vi "古田户外一体站流程质控自动启动.vi"(11 "参数":T1={"是否启用仪器"=FALSE, "CODMn"={"启动测量模式"={"测量模式"=enum."水样测量"}, "确定按钮"=TRUE}, "启动模块"={"氨氮"=FALSE, "总磷"=FALSE, "总氮"=FALSE, "COD"=FALSE}, "常规启动"=FALSE, "直接启动"=FALSE}) -> ()   [LabVIEW 2016, in "质控单元.lvlib"]
uses:
  PLC/PLC.lvlib
panel:
  out "枚举 2":enum16{"初始化", "采配水启动", "等待", "配水", "排水", "结束"}(ring)
  out "枚举":enum16{"初始化", "采配水启动", "等待", "配水", "排水", "结束"}(ring)
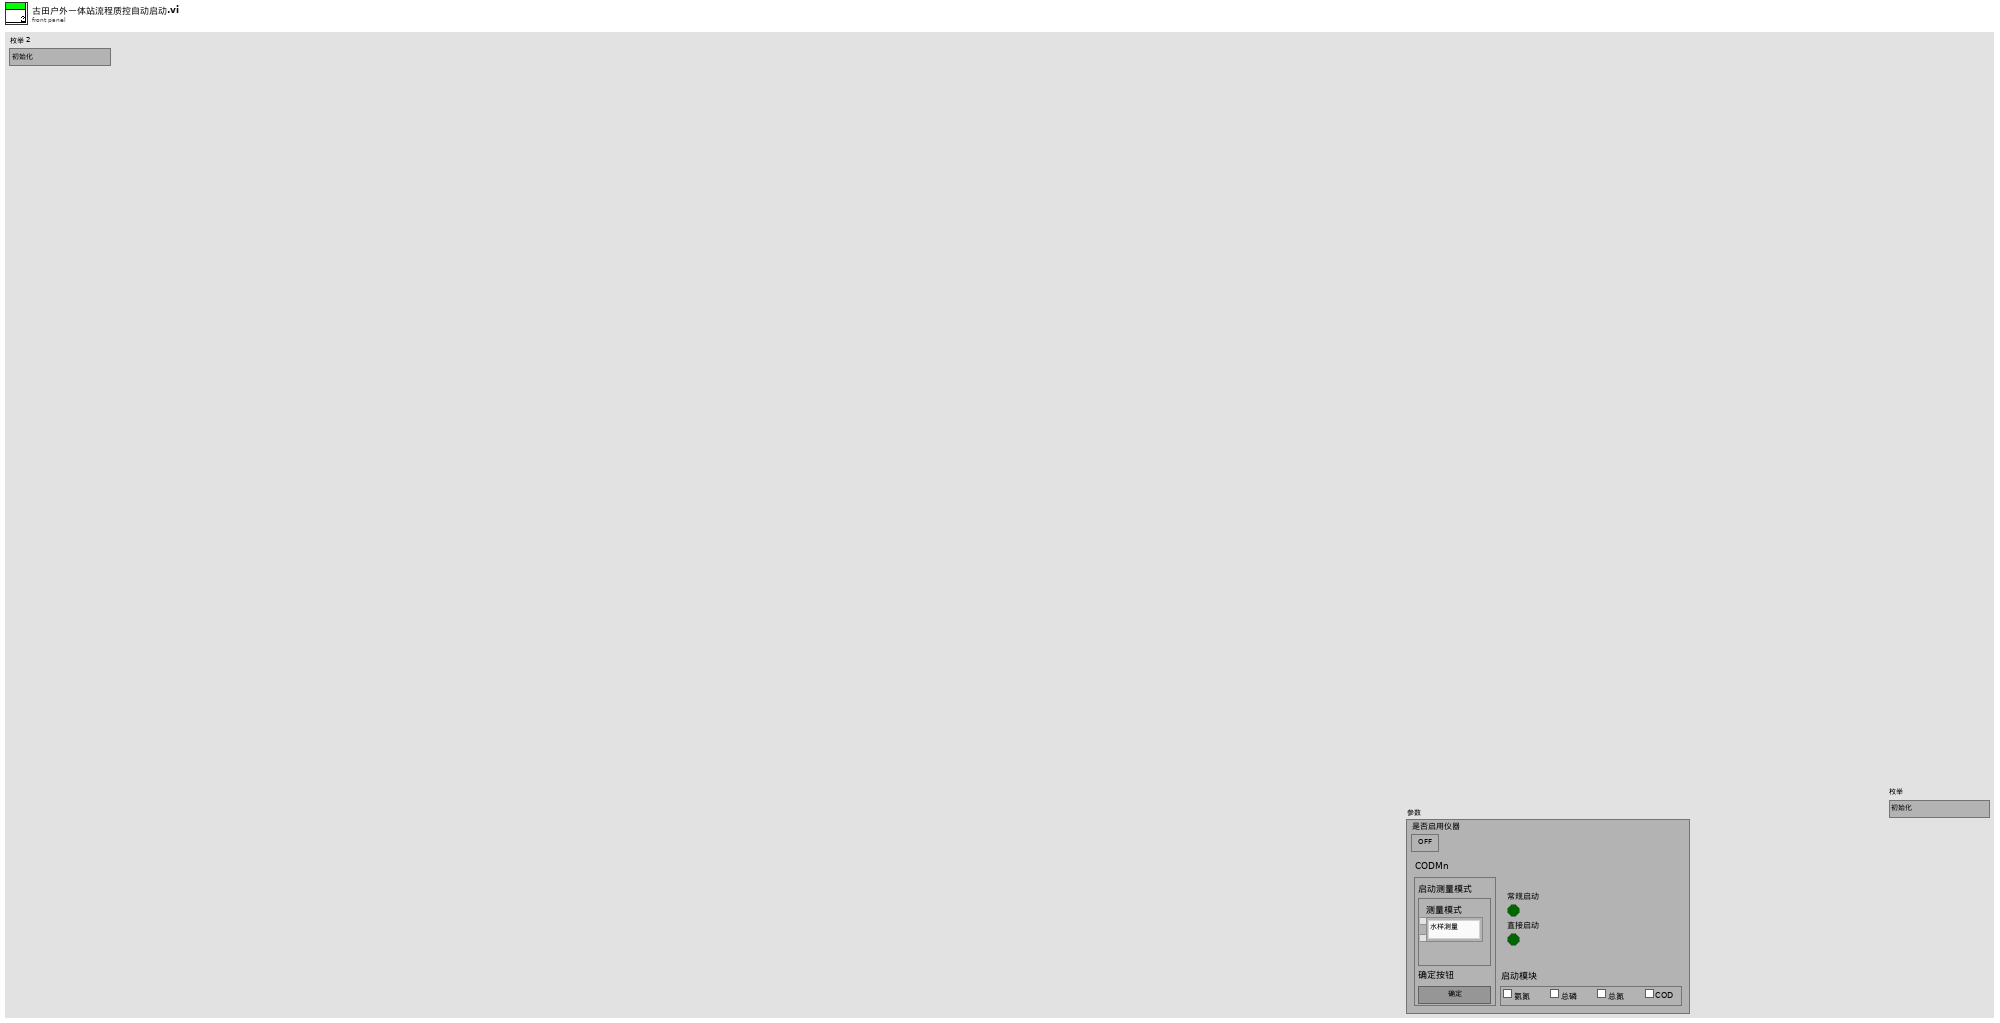
[diagram p1: front panel]
types:
  T1 = cluster{"是否启用仪器":bool, "CODMn":cluster{"启动测量模式":cluster{"测量模式":enum16{"水样测量", "标样核查", "加标回收", "平行样", "校零", "校标"}}, "确定按钮":bool}, "启动模块":cluster{"氨氮":bool, "总磷":bool, "总氮":bool, "COD":bool}, "常规启动":bool, "直接启动":bool}
  T2 = cluster{"命令":string, cluster{"starting address":u16, "holding register value":u16}}
  T3 = cluster{"R0":i16, "R1":i16, "R2":i16, "R3":i16, "R4":i16, "R5":i16, "R6":i16, "R7":i16, "R8":i16, "R9":i16, "R10":i16, "R11":i16, "R12":i16, "R13":i16, "R14":i16, "R15":i16, "R16":i16, "R17":i16, "R18":i16, "R19":i16, "R20":i16, "R21":i16}
  T4 = enum32{"Bad", "Idle", "Run top level", "Running"}
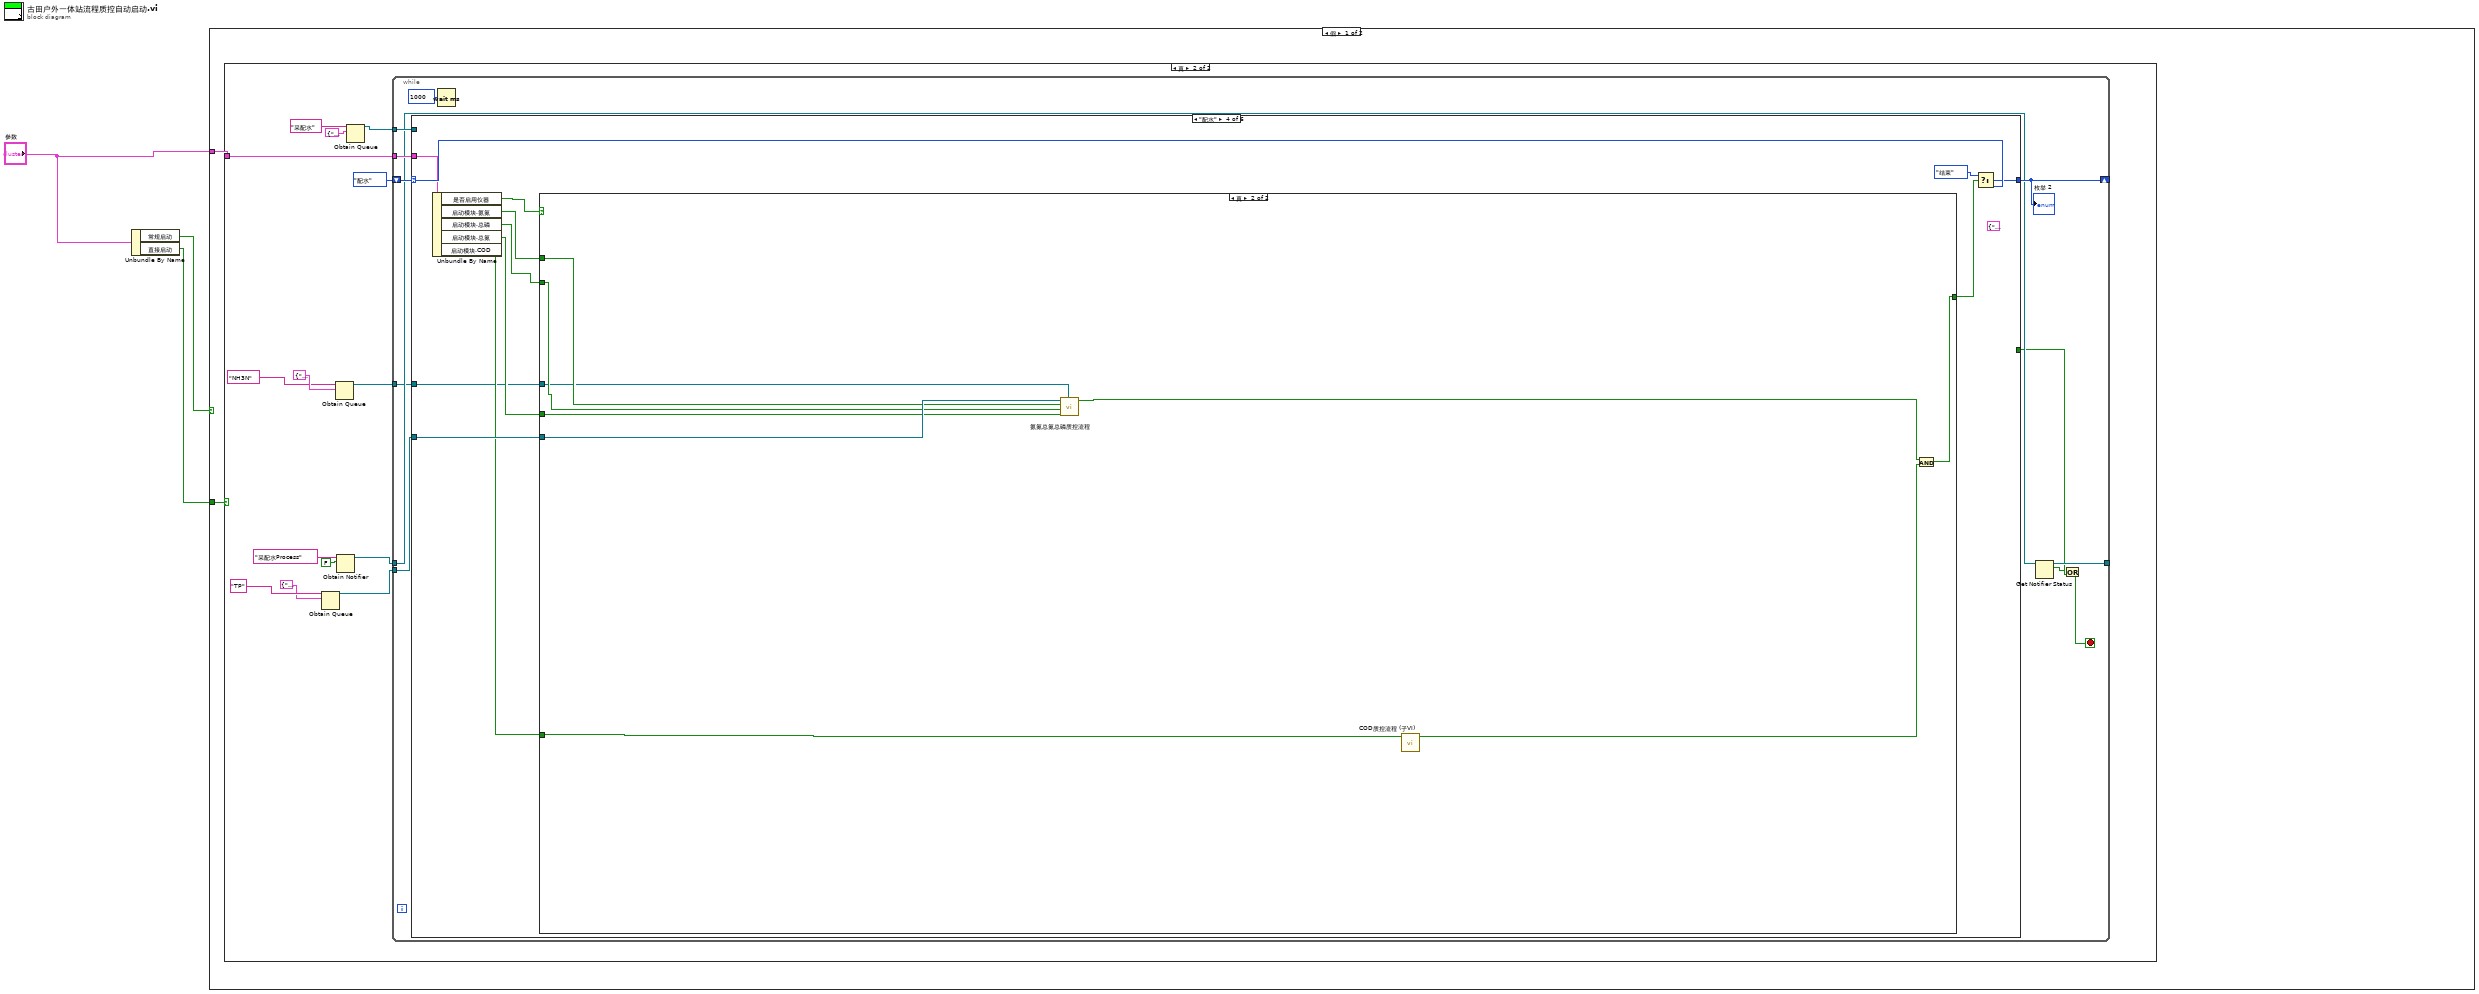
[diagram p0: block diagram]
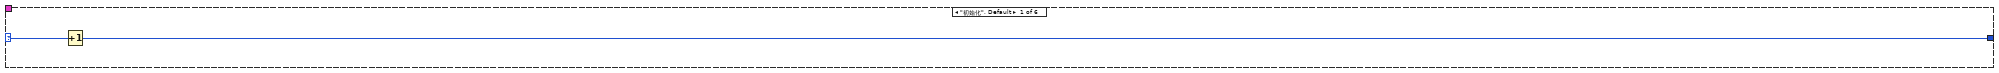
[diagram p3: hidden frame]
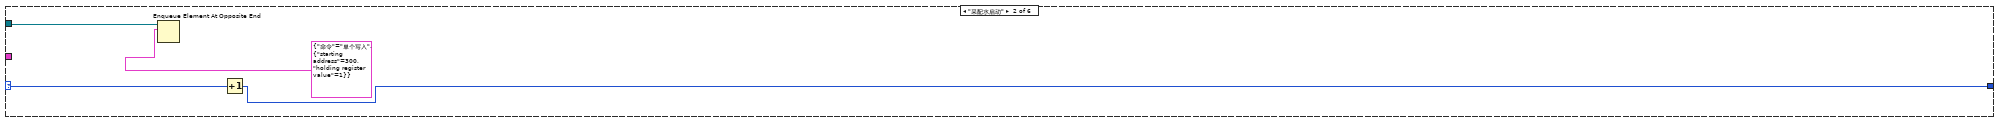
[diagram p4: hidden frame]
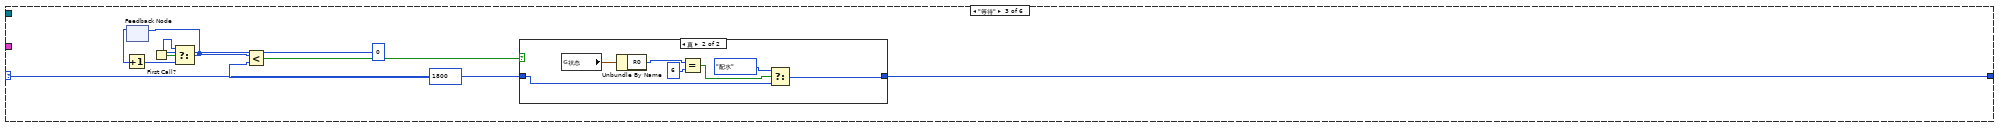
[diagram p5: hidden frame]
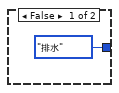
[diagram p6: hidden frame]
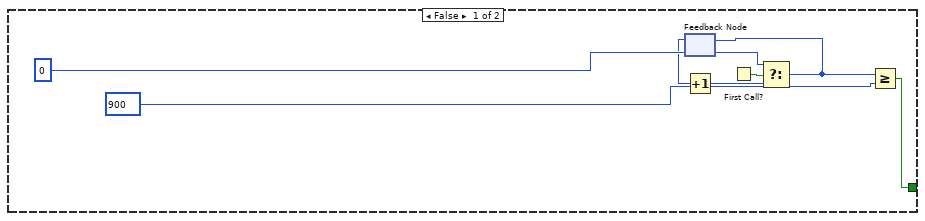
[diagram p7: hidden frame]
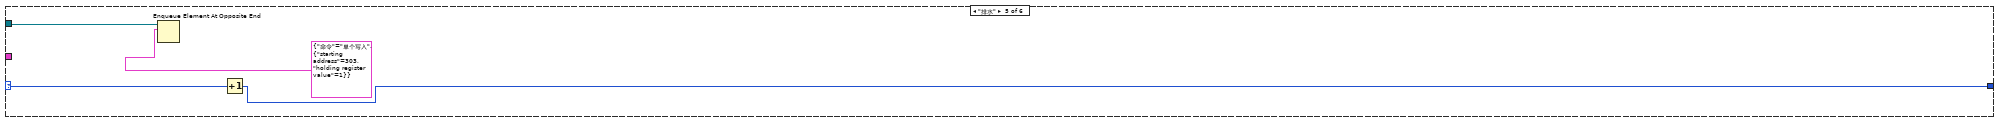
[diagram p8: hidden frame]
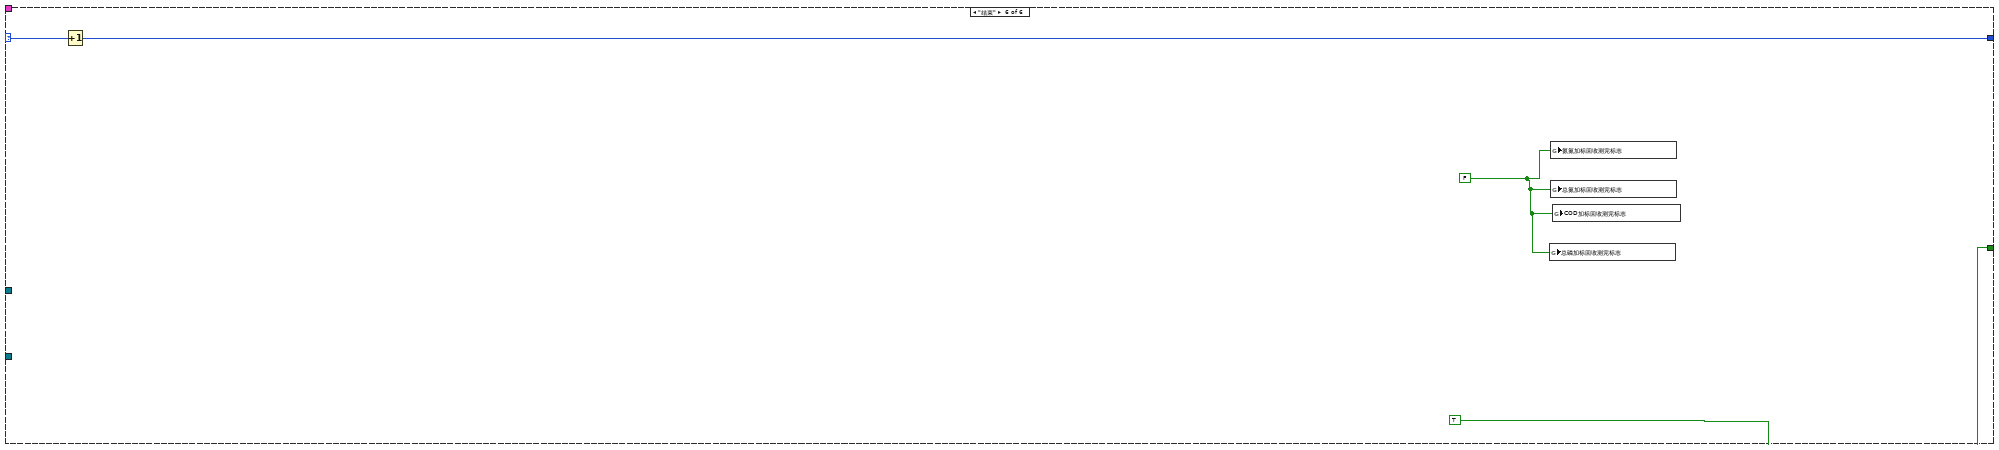
[diagram p9: hidden frame]
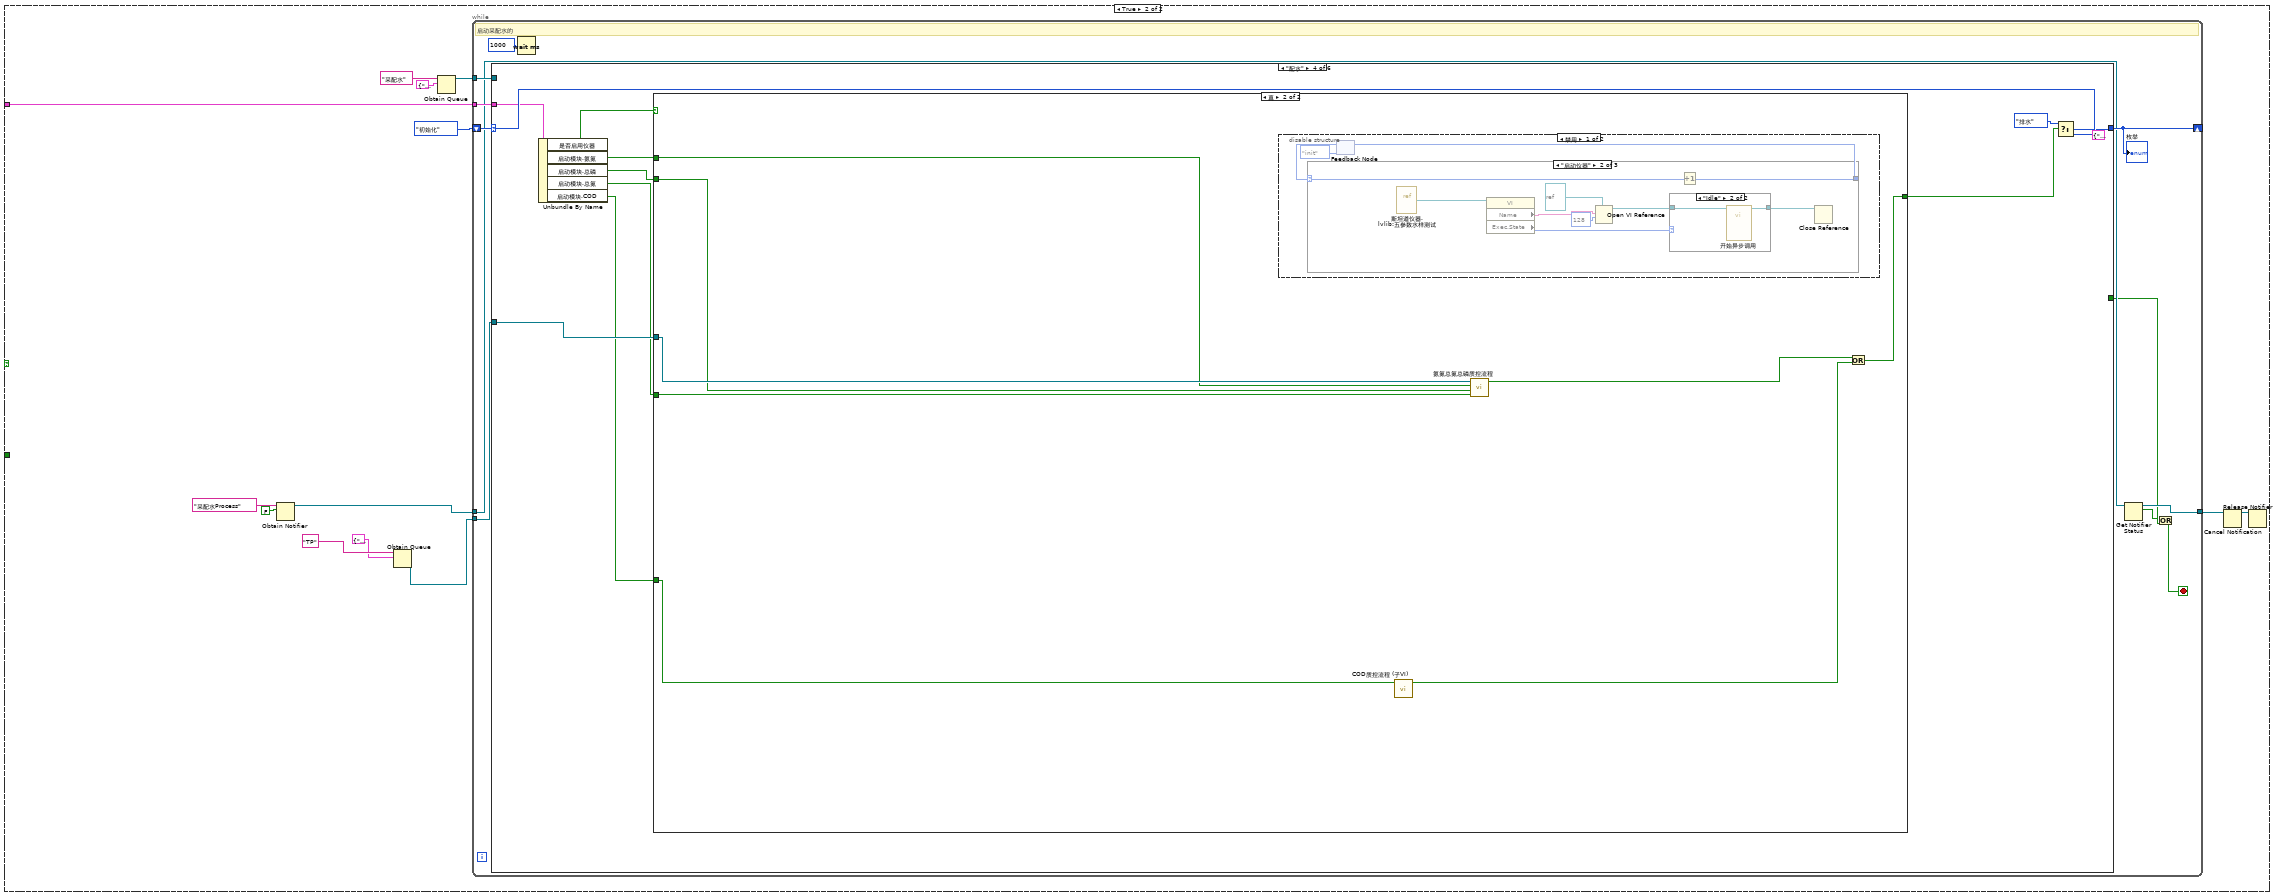
[diagram p10: hidden frame]
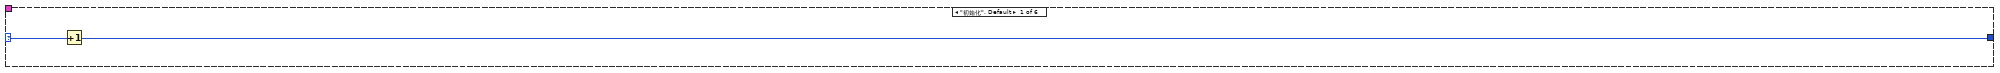
[diagram p11: hidden frame]
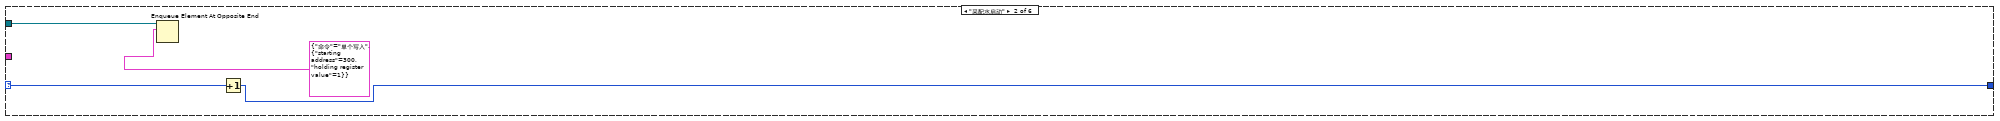
[diagram p12: hidden frame]
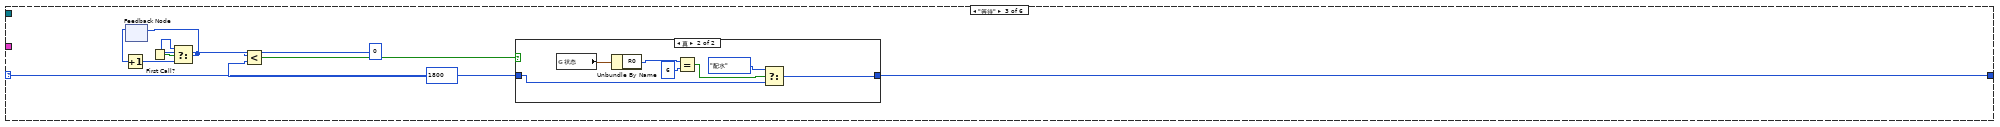
[diagram p13: hidden frame]
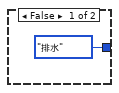
[diagram p14: hidden frame]
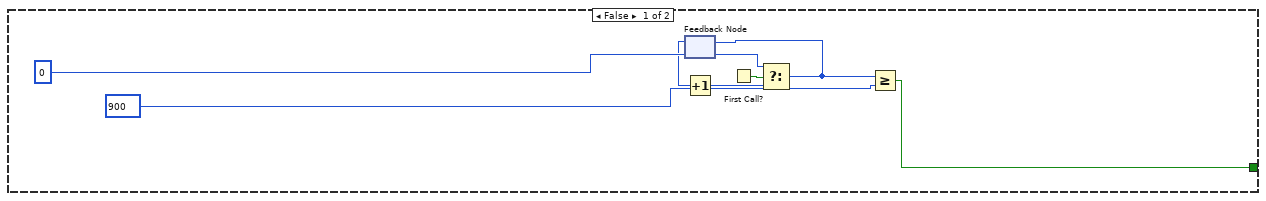
[diagram p15: hidden frame]
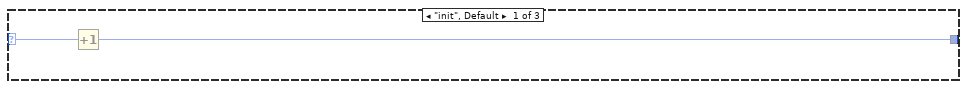
[diagram p16: hidden frame]
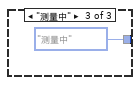
[diagram p18: hidden frame]
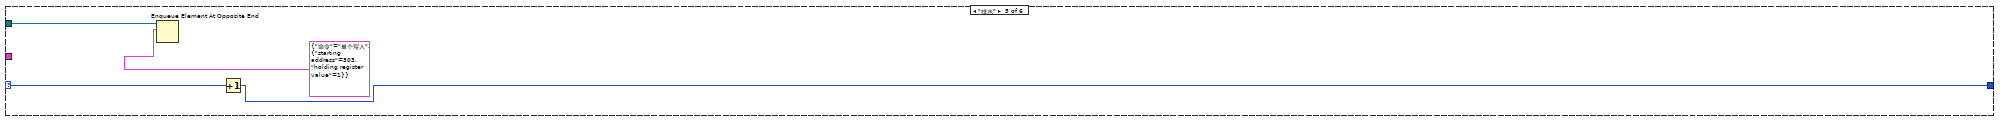
[diagram p20: hidden frame]
diagram:
  n1 = Unbundle By Name("参数") -> ("常规启动"=w2:bool, "直接启动"=w1:bool)
  n2 = case shown="假" w2 {
    tunnel: "参数" -> [w4 w91]
    tunnel: w1 -> [w5 _]
    frame False {
      n3 = case shown="真" w5 {
        tunnel: w4 -> [_ w18]
        frame False {
        }
        frame True {
          n4 = Obtain Queue(name (unnamed)="TP" ("名称（未命名）"), element data type=cluster{"命令":string, "data":variant} {"命令"="", "data"=variant}) -> (queue out=w9:refnum<queue>)  [unwired: 3 in, 2 out]
          n5 = Obtain Queue(name (unnamed)="NH3N" ("名称（未命名）"), element data type=cluster{"命令":string, "data":variant} {"命令"="", "data"=variant}) -> (queue out=w6:refnum<queue>)  [unwired: 3 in, 2 out]
          n6 = Obtain Notifier(name (unnamed)="采配水Process" ("名称（未命名）"), notification data type=FALSE) -> (notifier out=w12:refnum<notifier>)  [unwired: 2 in, 2 out]
          n7 = Obtain Queue(name (unnamed)="采配水" ("名称（未命名）"), element data type=cluster{"命令":string, "数据":variant} {"命令"="", "数据"=variant}) -> (queue out=w15:refnum<queue>)  [unwired: 3 in, 2 out]
          n8 = while {
            tunnel: w15 -> [w31]
            shift-right: [w29] -> _
            shift-left: enum16{"初始化", "采配水启动", "等待", "配水", "排水", "结束"}."配水" ("枚举") -> [w30]
            tunnel: w9 -> [w27]
            tunnel: w18 -> [w26]
            tunnel: w12 -> [w25]
            tunnel: [w24] -> _
            tunnel: w6 -> [w20]
            stop <- w23 stop-if-true
            n9 = case shown="\"配水\"" w30 {
              selector: w30 -> [w33 w35 w44 w65 w84 w90]
              tunnel: w31 -> [_ w36 _ _ w85 _]
              tunnel: [w32 w34 w43 w64 w83 w89] -> w29
              tunnel: [_ _ _ _ _ TRUE] -> w22
              tunnel: w27 -> [_ _ _ w63 _ _]
              tunnel: w26 -> [_ _ _ w60 _ _]
              tunnel: w20 -> [_ _ _ w55 _ _]
              frame "初始化", Default {
                n10 = Increment(x=w33) -> (x+1=w32:enum16{"初始化", "采配水启动", "等待", "配水", "排水", "结束"})
              }
              frame "采配水启动" {
                n11 = Enqueue Element At Opposite End(queue=w36, element=T2 {"命令"="单个写入", {"starting address"=300, "holding register value"=1}} ("元素")) -> ()  [unwired: 2 in, 3 out]
                n12 = Increment(x=w35) -> (x+1=w34:enum16{"初始化", "采配水启动", "等待", "配水", "排水", "结束"})
              }
              frame "等待" {
                n13 = feedback #1() -> (w40:i32)  [unwired: 1 in]
                n14 = Increment(x=w40) -> (x+1=w39:i32)
                n15 = First Call?() -> (First Call?: T/F=w41:bool)
                n16 = Select(t=0, s=w41, f=w39) -> (s? t:f=w38:i32)
                n17 = feedback-in #1(w38) -> ()
                n18 = Less?(x=w38, y=1800) -> (x < y?=w45:bool)
                n19 = case shown="真" w45 {
                  tunnel: w44 -> [_ w49]
                  tunnel: [enum16{"初始化", "采配水启动", "等待", "配水", "排水", "结束"}."排水" ("枚举") w48] -> w43
                  frame False {
                  }
                  frame True {
                    n20 = global read "采配水全局变量.vi" "状态"() -> (w54:T3)
                    n21 = Unbundle By Name(w54) -> ("R0"=w53:i16)
                    n22 = Equal?(x=w53, y=i16 6) -> (x = y?=w51:bool)
                    n23 = Select(t=enum16{"初始化", "采配水启动", "等待", "配水", "排水", "结束"}."配水" ("枚举"), s=w51, f=w49) -> (s? t:f=w48:enum16{"初始化", "采配水启动", "等待", "配水", "排水", "结束"})
                  }
                }
              }
              frame "配水" {
                (unwired) cluster{"命令":string, "data":variant} {"命令"="启动", "data"=variant(cluster{"站号":u16, "控制命令输出":u16[]} {"站号"=1, "控制命令输出"=[256, 0]})} ("元素")
                n24 = Unbundle By Name(w60) -> ("是否启用仪器"=w62:bool, "启动模块.氨氮"=w58:bool, "启动模块.总磷"=w59:bool, "启动模块.总氮"=w56:bool, "启动模块.COD"=w57:bool)
                n25 = case shown="真" w62 {
                  tunnel: w63 -> [_ w81]
                  tunnel: [w67 w82] -> w61
                  tunnel: w59 -> [_ w79]
                  tunnel: w58 -> [_ w80]
                  tunnel: w57 -> [_ w78]
                  tunnel: w56 -> [_ w75]
                  tunnel: w55 -> [_ w74]
                  frame False {
                    n26 = feedback #2() -> (w71:i32)  [unwired: 1 in]
                    n27 = Increment(x=w71) -> (x+1=w70:i32)
                    n28 = First Call?() -> (First Call?: T/F=w72:bool)
                    n29 = Select(t=0, s=w72, f=w70) -> (s? t:f=w68:i32)
                    n30 = feedback-in #2(w68) -> ()
                    n31 = Greater Or Equal?(x=w68, y=900) -> (x >= y?=w67:bool)
                  }
                  frame True {
                    n32 = call "氨氮总氮总磷质控流程.vi"("队列输入NH3"=w74, "总氮"=w75, "总磷"=w79, "氨氮"=w80, "队列输入TP"=w81) -> ("布尔"=w76:bool)  [unwired: 6 in]
                    n33 = call "COD质控流程 (子VI).vi"("COD"=w78) -> ("布尔"=w77:bool)  [unwired: 10 in]
                    n34 = And(x=w76, y=w77) -> (x .and. y?=w82:bool)
                  }
                }
                n35 = Select(t=enum16{"初始化", "采配水启动", "等待", "配水", "排水", "结束"}."结束" ("枚举"), s=w61, f=w65) -> (s? t:f=w64:enum16{"初始化", "采配水启动", "等待", "配水", "排水", "结束"})
              }
              frame "排水" {
                n36 = Enqueue Element At Opposite End(queue=w85, element=T2 {"命令"="单个写入", {"starting address"=303, "holding register value"=1}} ("元素")) -> ()  [unwired: 2 in, 3 out]
                n37 = Increment(x=w84) -> (x+1=w83:enum16{"初始化", "采配水启动", "等待", "配水", "排水", "结束"})
              }
              frame "结束" {
                w87 = FALSE ("氨氮加标回收测完标志")
                n38 = Increment(x=w90) -> (x+1=w89:enum16{"初始化", "采配水启动", "等待", "配水", "排水", "结束"})
                n39 = global write "质控测完标志全局 1.vi" "总磷加标回收测完标志"(w87) -> ()
                n40 = global write "质控测完标志全局 1.vi" "氨氮加标回收测完标志"(w87) -> ()
                n41 = global write "质控测完标志全局 1.vi" "总氮加标回收测完标志"(w87) -> ()
                n42 = global write "质控测完标志全局 1.vi" "COD加标回收测完标志"(w87) -> ()
              }
            }
            "枚举 2" <- w29
            n43 = Wait (ms)(milliseconds to wait=u32 1000 ("等待时间（毫秒）")) -> ()  [unwired: 1 out]
            n44 = Get Notifier Status(notifier=w25) -> (notifier out=w24:refnum<notifier>, current notification=w21:bool)  [unwired: 1 in, 3 out]
            n45 = Or(x=w21, y=w22) -> (x .or. y?=w23:bool)
          }
        }
      }
    }
    frame True {
      n46 = Obtain Notifier(name (unnamed)="采配水Process" ("名称（未命名）"), notification data type=FALSE) -> (notifier out=w94:refnum<notifier>)  [unwired: 2 in, 2 out]
      n47 = Obtain Queue(name (unnamed)="TP" ("名称（未命名）"), element data type=cluster{"命令":string, "data":variant} {"命令"="", "data"=variant}) -> (queue out=w97:refnum<queue>)  [unwired: 3 in, 2 out]
      n48 = Obtain Queue(name (unnamed)="采配水" ("名称（未命名）"), element data type=cluster{"命令":string, "数据":variant} {"命令"="", "数据"=variant}) -> (queue out=w101:refnum<queue>)  [unwired: 3 in, 2 out]
      n49 = while {
        tunnel: w101 -> [w114]
        shift-right: [w112] -> _
        shift-left: enum16{"初始化", "采配水启动", "等待", "配水", "排水", "结束"}."初始化" ("枚举") -> [w113]
        tunnel: w97 -> [w110]
        tunnel: w91 -> [w109]
        tunnel: w94 -> [w108]
        tunnel: [w107] -> w93
        stop <- w106 stop-if-true
        # "启动采配水的"
        n50 = case shown="\"配水\"" w113 {
          selector: w113 -> [w116 w118 w127 w147 w183 w188]
          tunnel: w114 -> [_ w119 _ _ w184 _]
          tunnel: [w115 w117 w126 w146 w182 w187] -> w112
          tunnel: [_ _ _ _ _ TRUE] -> w105
          tunnel: w110 -> [_ _ _ w145 _ _]
          tunnel: w109 -> [_ _ _ w142 _ _]
          frame "初始化", Default {
            n51 = Increment(x=w116) -> (x+1=w115:enum16{"初始化", "采配水启动", "等待", "配水", "排水", "结束"})
          }
          frame "采配水启动" {
            n52 = Enqueue Element At Opposite End(queue=w119, element=T2 {"命令"="单个写入", {"starting address"=300, "holding register value"=1}} ("元素")) -> ()  [unwired: 2 in, 3 out]
            n53 = Increment(x=w118) -> (x+1=w117:enum16{"初始化", "采配水启动", "等待", "配水", "排水", "结束"})
          }
          frame "等待" {
            n54 = feedback #3() -> (w123:i32)  [unwired: 1 in]
            n55 = Increment(x=w123) -> (x+1=w122:i32)
            n56 = First Call?() -> (First Call?: T/F=w124:bool)
            n57 = Select(t=0, s=w124, f=w122) -> (s? t:f=w121:i32)
            n58 = feedback-in #3(w121) -> ()
            n59 = Less?(x=w121, y=1800) -> (x < y?=w128:bool)
            n60 = case shown="真" w128 {
              tunnel: w127 -> [_ w132]
              tunnel: [enum16{"初始化", "采配水启动", "等待", "配水", "排水", "结束"}."排水" ("枚举") w131] -> w126
              frame False {
              }
              frame True {
                n61 = global read "采配水全局变量.vi" "状态"() -> (w137:T3)
                n62 = Unbundle By Name(w137) -> ("R0"=w136:i16)
                n63 = Equal?(x=w136, y=i16 6) -> (x = y?=w134:bool)
                n64 = Select(t=enum16{"初始化", "采配水启动", "等待", "配水", "排水", "结束"}."配水" ("枚举"), s=w134, f=w132) -> (s? t:f=w131:enum16{"初始化", "采配水启动", "等待", "配水", "排水", "结束"})
              }
            }
          }
          frame "配水" {
            (unwired) cluster{"命令":string, "data":variant} {"命令"="启动", "data"=variant(cluster{"站号":u16, "控制命令输出":u16[]} {"站号"=1, "控制命令输出"=[256, 0]})} ("元素")
            n65 = Unbundle By Name(w142) -> ("是否启用仪器"=w144:bool, "启动模块.氨氮"=w140:bool, "启动模块.总磷"=w141:bool, "启动模块.总氮"=w138:bool, "启动模块.COD"=w139:bool)
            n66 = case shown="真" w144 {
              tunnel: w145 -> [_ w163]
              tunnel: [w149 w160] -> w143
              tunnel: w141 -> [_ w159]
              tunnel: w140 -> [_ w158]
              tunnel: w139 -> [_ w157]
              tunnel: w138 -> [_ w156]
              frame False {
                n67 = feedback #4() -> (w153:i32)  [unwired: 1 in]
                n68 = Increment(x=w153) -> (x+1=w152:i32)
                n69 = First Call?() -> (First Call?: T/F=w154:bool)
                n70 = Select(t=0, s=w154, f=w152) -> (s? t:f=w150:i32)
                n71 = feedback-in #4(w150) -> ()
                n72 = Greater Or Equal?(x=w150, y=900) -> (x >= y?=w149:bool)
              }
              frame True {
                n73 = disable-structure shown="禁用" {
                  frame Disabled {
                    n74 = feedback #5(enum16{"init", "启动仪器", "测量中"}."init") -> (w165:enum16{"init", "启动仪器", "测量中"})
                    n75 = case shown="\"启动仪器\"" w165 {
                      selector: w165 -> [w168 w177 _]
                      tunnel: [w167 w176 enum16{"init", "启动仪器", "测量中"}."测量中"] -> w166
                      frame "init", Default {
                        n76 = Increment(x=w168) -> (x+1=w167:enum16{"init", "启动仪器", "测量中"})
                      }
                      frame "启动仪器" {
                        n77 = vi-ref "斯坦道仪器.lvlib:五参数水样测试.vi"() -> (w169:refnum<vi>)
                        n78 = property class="VI"(reference=w169) -> ("Name"=w173:string, "Exec.State"=w171:T4)  [unwired: 1 in, 2 out]
                        n79 = Open VI Reference(type specifier VI Refnum (for type only)=refnum<vi> refnum ("类型说明符VI引用句柄（仅用于类型）"), vi path=w173, options=128 ("选项")) -> (vi reference=w172:refnum<vi>)  [unwired: 3 in, 1 out]
                        n80 = case shown="\"Idle\"" w171 {
                          tunnel: w172 -> [w178 w180]
                          tunnel: [w178 w179] -> w170
                          frame "Bad", Default {
                          }
                          frame "Idle" {
                            n81 = call-by-ref "开始异步调用"(reference=w180) -> (reference out=w179:refnum<vi>)  [unwired: 13 in, 1 out]
                          }
                        }
                        n82 = Increment(x=w177) -> (x+1=w176:enum16{"init", "启动仪器", "测量中"})
                        n83 = Close Reference(reference=w170) -> ()  [unwired: 1 in, 1 out]
                      }
                      frame "测量中" {
                      }
                    }
                    n84 = feedback-in #5(w166) -> ()
                  }
                  frame Enabled {
                  }
                }
                n85 = call "COD质控流程 (子VI).vi"("COD"=w157) -> ("布尔"=w161:bool)  [unwired: 10 in]
                n86 = call "氨氮总氮总磷质控流程.vi"("总氮"=w156, "总磷"=w159, "氨氮"=w158, "队列输入TP"=w163) -> ("布尔"=w162:bool)  [unwired: 7 in]
                n87 = Or(x=w162, y=w161) -> (x .or. y?=w160:bool)
              }
            }
            n88 = Select(t=enum16{"初始化", "采配水启动", "等待", "配水", "排水", "结束"}."排水" ("枚举"), s=w143, f=w147) -> (s? t:f=w146:enum16{"初始化", "采配水启动", "等待", "配水", "排水", "结束"})
          }
          frame "排水" {
            n89 = Enqueue Element At Opposite End(queue=w184, element=T2 {"命令"="单个写入", {"starting address"=303, "holding register value"=1}} ("元素")) -> ()  [unwired: 2 in, 3 out]
            n90 = Increment(x=w183) -> (x+1=w182:enum16{"初始化", "采配水启动", "等待", "配水", "排水", "结束"})
          }
          frame "结束" {
            n91 = Increment(x=w188) -> (x+1=w187:enum16{"初始化", "采配水启动", "等待", "配水", "排水", "结束"})
          }
        }
        "枚举" <- w112
        n92 = Wait (ms)(milliseconds to wait=u32 1000 ("等待时间（毫秒）")) -> ()  [unwired: 1 out]
        n93 = Get Notifier Status(notifier=w108) -> (notifier out=w107:refnum<notifier>, current notification=w104:bool)  [unwired: 1 in, 3 out]
        n94 = Or(x=w104, y=w105) -> (x .or. y?=w106:bool)
      }
      n95 = Cancel Notification(0:w93) -> (8:w92:refnum<notifier>)  [unwired: 1 in, 2 out]
      n96 = Release Notifier(notifier=w92) -> ()  [unwired: 2 in, 3 out]
    }
  }
